vi "Untitled 1.vi"() -> ()   [LabVIEW 2013]
panel:
  out "conf col":i32
  in  "unit to search for":u16
  out "number":u16[](array[numeric])
  in  "Formulas definitions":string[][](table)=[["CO ppm", "3*x"], ["O2 %", "-20*x"]]
  in  "Application-specific conversion settings":T1 {"Fxn array names 2" items=[".", "O2 %", "CO ppm", "new"]}
  in  "Unit conf cat.":string[](array[string])
  in  "stop":bool
  in  "Fxn array names":u16[][](array[ring]) items=[".", "O2 %", "CO ppm", "new"]
  # "Comma separated unit selection (default keyword for others)"
  # "Convertion formulas definition"
  # "A1.0"
  # "A1.1"
  # "Formula name[units]"
  # "Formula definition"
  # "A1.2"
  # "A1.3"
  # "A2.0"
  # "A2.1"
  # "A2.2"
  # "A2.3"
  # "A3.0"
  # "A3.1"
  # "A3.2"
  # "A3.3"
  # "no spaces!"
  # "no commas!"
  # "Comma separated unit selection (default keyword for others)"
  # "A1.0"
  # "A1.1"
  # "A1.2"
  # "A1.3"
  # "A2.0"
  # "A2.1"
  # "A2.2"
  # "A2.3"
  # "A3.0"
  # "A3.1"
  # "A3.2"
  # "A3.3"
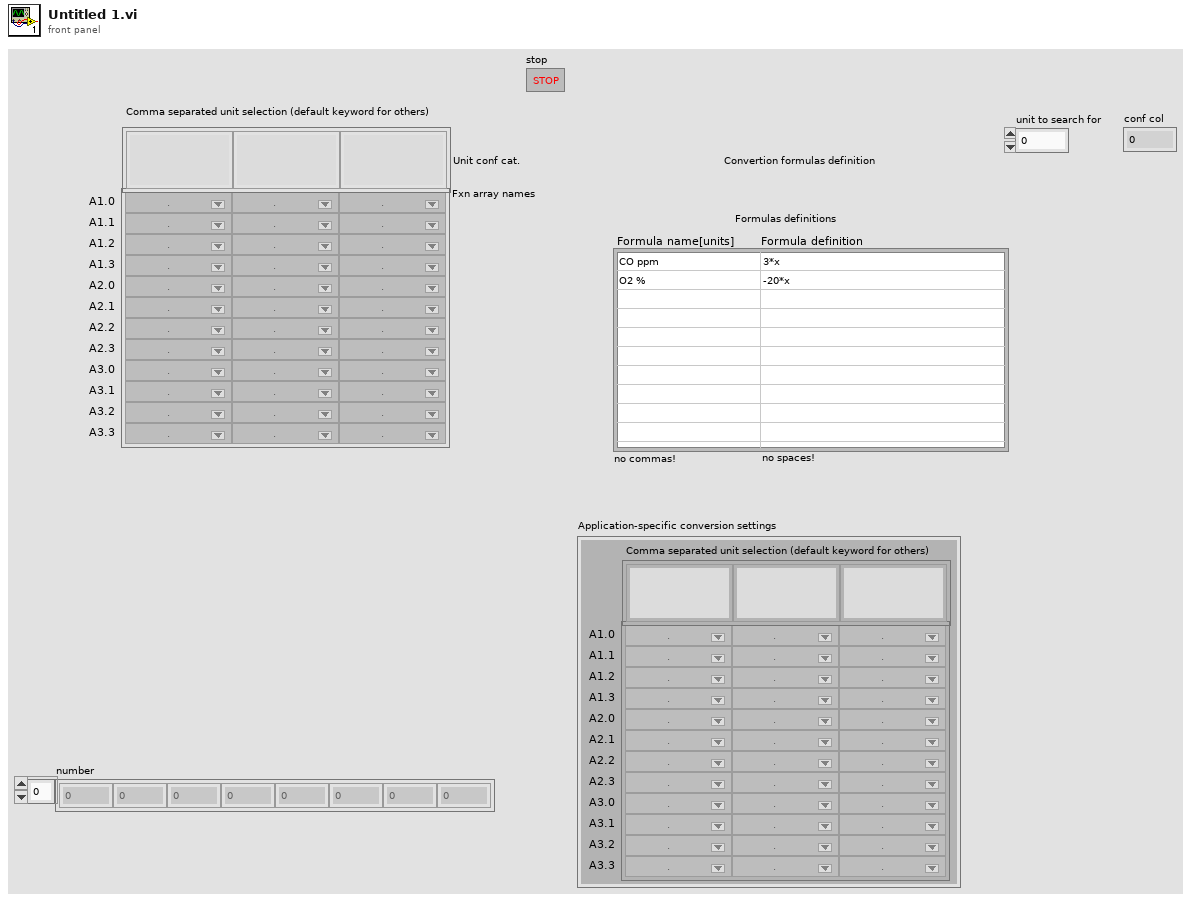
[diagram p1: front panel]
types:
  T1 = cluster{"Fxn array names 2":u16[][], "Unit conf cat. 2":string[]}
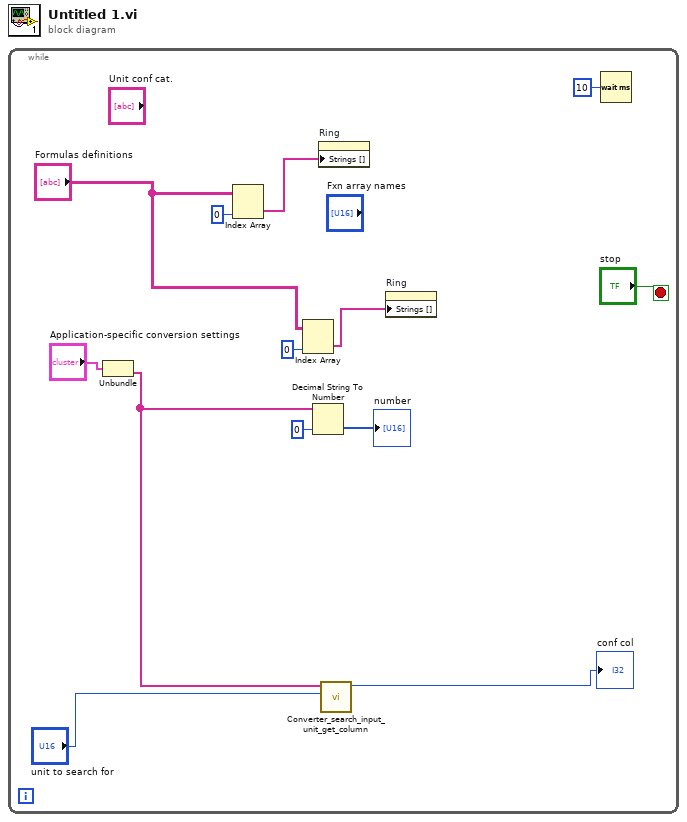
[diagram p0: block diagram]
diagram:
  n1 = while {
    stop <- "stop" stop-if-true
    n2 = Unbundle("Application-specific conversion settings") -> ("Unit conf cat. 2"=w3:string[])  [unwired: 1 out]
    n3 = Index Array(array="Formulas definitions", index (col)=0 ("disabled index (col)")) -> (element=w12:string[])  [unwired: 1 in]
    n4 = Index Array(array="Formulas definitions", index (col)=0 ("disabled index (col)")) -> (element=w8:string[])  [unwired: 1 in]
    n5 = Decimal String To Number(string=w3, default (0L)=u16 0 ("default (0 I32)")) -> (number=→"number":u16[])  [unwired: 1 in, 1 out]
    n6 = property on="Ring" class="Ring (strict)"("Strings []"=w12) -> ()  [unwired: 2 in, 2 out]
    n7 = call "Converter_search_input_unit_get_column.vi"("unit to search for"="unit to search for", "Unit conf cat. in"=w3) -> ("found in column number"=→"conf col":i32)  [unwired: 9 in]
    n8 = property on="Ring" class="Ring (strict)"("Strings []"=w8) -> ()  [unwired: 2 in, 2 out]
    n9 = Wait (ms)(milliseconds to wait=u32 10) -> ()  [unwired: 1 out]
  }
